vi "ZXing Read Barcodes (Greyscale All).vi"(8 "error in (no error)":errorcluster, 11 "Greyscale Image in":T1) -> (0 "error out":errorcluster, 3 "Greyscale Image":T1)   [LabVIEW 2020, in "feature_detection.lvlib"]
doc: "Finds contours in a binary image. Detected contours can be further processed using functions such as Approximate Polygon.vi and Contour Conver Hull.vi."
uses:
  feature_detection.lvlib
  image/Greyscale Image.ctl
  common/common.lvlib
  common/bin/gartoolkit_32-1.dll
  image/image.lvlib
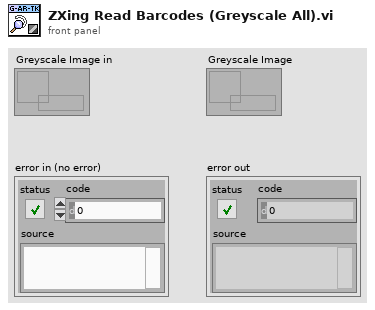
[diagram p1: front panel]
types:
  T1 = typedef "image.lvlib/Greyscale Image.ctl" = refnum<data-value>
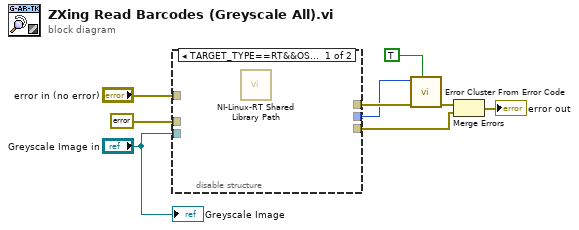
[diagram p0: block diagram]
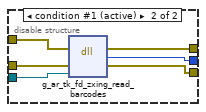
[diagram p2: hidden frame]
diagram:
  n1 = disable-structure shown="TARGET_TYPE==RT&&OS==Linux" {
    disable-tunnel: "error in (no error)" -> [_ w15]
    disable-tunnel: errorcluster {"status"=FALSE, "code"=0, "source"=""} ("error constant") -> [_ w14]
    disable-tunnel: "Greyscale Image in" -> [_ w13]
    disable-tunnel: [_ w12] -> w4
    disable-tunnel: [_ w11] -> w3
    disable-tunnel: [_ w10] -> w2
    frame condition #0 {
      n2 = call "NI-Linux-RT Shared Library Path.vi"() -> ()  [unwired: 1 out]
    }
    frame condition #1 (active) {
      n3 = dll-call lib="C:/serenial/lib/g-augmented-reality-toolkit/LabVIEW/common/bin/gartoolkit_*-1.*" fn="g_ar_tk_fd_zxing_read_barcodes" ("g_ar_toolkit.*.*:g_ar_tk_image_draw_line")(error in=w15, "error_cluster"=w14, "EDVR src"=w13) -> (error out=w12:errorcluster, "return type"=w11:i32, "error_cluster"=w10:errorcluster)  [unwired: 3 in, 1 out]
    }
  }
  n4 = call <vilib>:"Error Cluster From Error Code.vi"("show call chain? (False)"=TRUE, "error in (no error)"=w4, "error code (0)"=w3) -> ("error out"=w8:errorcluster)  [unwired: 6 in]
  n5 = Merge Errors(w8, w2) -> (→"error out":errorcluster)
  "Greyscale Image" <- "Greyscale Image in"
